vi "ACDC_Config.vi"(8 "error in (no error)":errorcluster, 9 "Input Config Array":T1[](array[typedef])=[0, 0, 0, 0, 0, 0, 0, 0, 0, 0, 0, 0, 0, 0, 0, 0, 0, 0, 0, 0, 0, 0, 0, 0, 0, 0, 0, 0, 0, 0, 0, 0] items=["AC Coupled", "DC Coupled", "IEPE AC Coupled"], 10 "Data Rate [S/s]":u32) -> (0 "error out":errorcluster)   [LabVIEW 2017, in "BOP_VibAPI_8.lvlib"]
uses:
  <vilib>/addons/InsightCM/Devices/Shared/Cms/Fpga/Acquisition/source/subVIs/VibAPI_8/BOP_VibAPI_8.lvlib
  <vilib>/LabVIEW Targets/FPGA/cRIO/shared/nicrio_ModuleControls/nicrio_cRIO-9232_ConfigModeRing.ctl
  <vilib>/rvi/eio/common/nirviEmuTemplatePropertySet_errors.vi
  <vilib>/eio/EIOPropertyNode/EIOPropertyNode.xnode
  <vilib>/LabVIEW Targets/FPGA/cRIO/shared/nicrio_ModuleControls/nicrio_cRIO-9232_DataRatesRing2.ctl
  <vilib>/rvi/eio/common/nirviEmuTemplatePropertyGet_errors.vi
  <vilib>/rvi/eio/common/nirviEmuTemplatePropertyGet_noerrors.vi
  <vilib>/rvi/eio/common/nirviEmuTemplatePropertySet_noerrors.vi
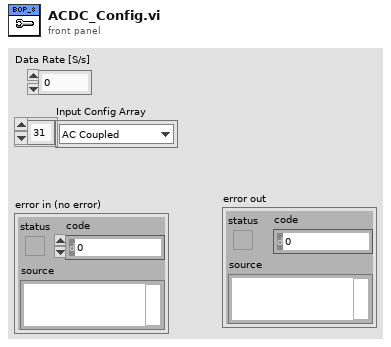
[diagram p1: front panel]
types:
  T1 = typedef "nicrio_cRIO-9232_ConfigModeRing.ctl" = u8
  T2 = typedef "nicrio_cRIO-9232_DataRatesRing2.ctl" = u8
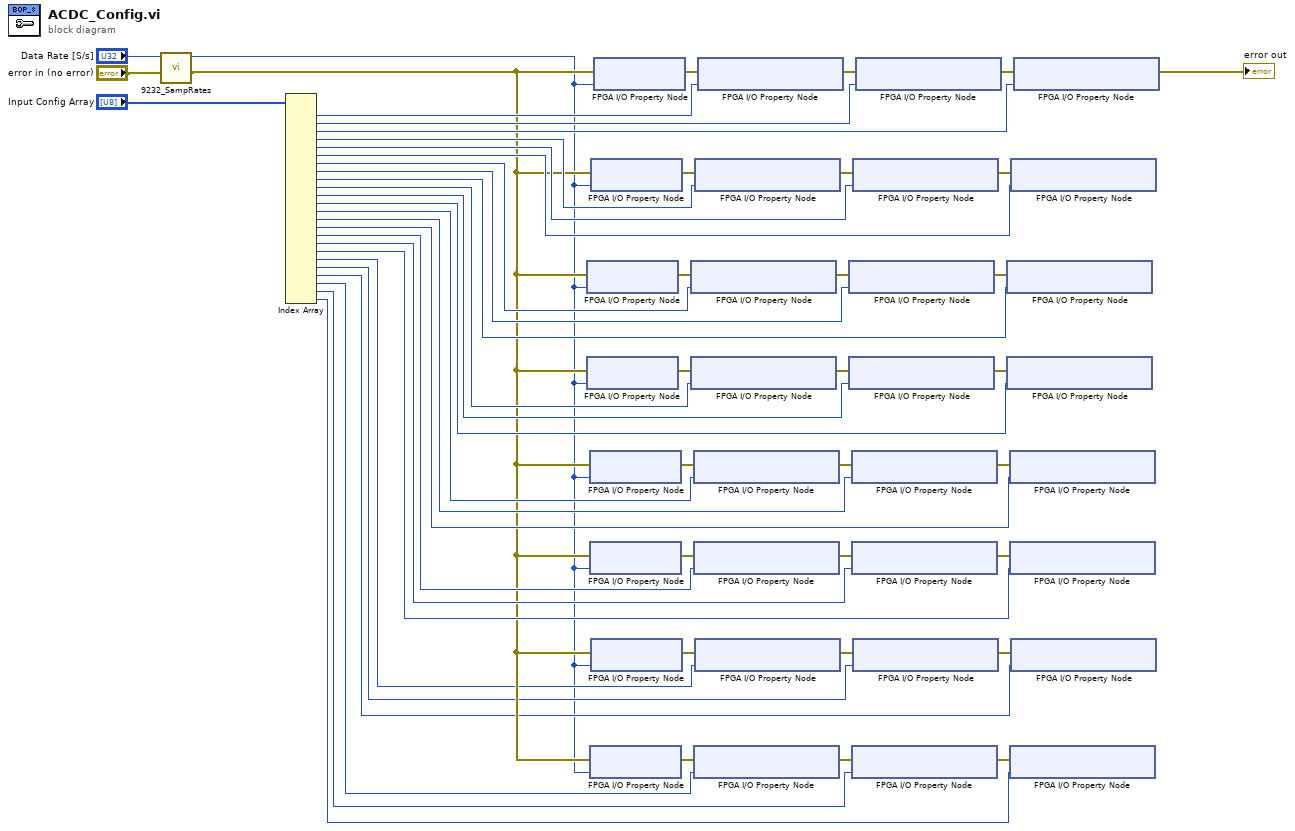
[diagram p0: block diagram]
diagram:
  n1 = call <vilib>:"9232_SampRates.vi"("error in (no error)"="error in (no error)", "Data Rate [S/s]"="Data Rate [S/s]") -> ("error out"=w8:errorcluster, "Data Rate"=w4:T2)  [unwired: 8 in]
  n2 = Index Array(array="Input Config Array") -> (element #1=w46:T1, element #2=w45:T1, element #3=w41:T1, element #4=w44:T1, element #5=w43:T1, element #6=w42:T1, element #7=w37:T1, element #8=w36:T1, element #9=w35:T1, element #10=w31:T1, element #11=w30:T1, element #12=w29:T1, element #13=w25:T1, element #14=w24:T1, element #15=w23:T1, element #16=w19:T1, element #17=w18:T1, element #18=w17:T1, element #19=w7:T1, element #20=w6:T1, element #21=w5:T1, element #22=w3:T1, element #23=w2:T1, element #24=w1:T1)  [unwired: 24 in]
  n3 = xnode "FPGA I/O Property Node"("error in"=w8, "Data Rate"=w4) -> ("error out"=w40:errorcluster)  [unwired: 1 in, 1 out]
  n4 = xnode "FPGA I/O Property Node"("error in"=w8, "Data Rate"=w4) -> ("error out"=w32:errorcluster)  [unwired: 1 in, 1 out]
  n5 = xnode "FPGA I/O Property Node"("error in"=w8, "Data Rate"=w4) -> ("error out"=w28:errorcluster)  [unwired: 1 in, 1 out]
  n6 = xnode "FPGA I/O Property Node"("error in"=w8, "Data Rate"=w4) -> ("error out"=w20:errorcluster)  [unwired: 1 in, 1 out]
  n7 = xnode "FPGA I/O Property Node"("error in"=w8, "Data Rate"=w4) -> ("error out"=w9:errorcluster)  [unwired: 1 in, 1 out]
  n8 = xnode "FPGA I/O Property Node"("error in"=w8, "Data Rate"=w4) -> ("error out"=w47:errorcluster)  [unwired: 1 in, 1 out]
  n9 = xnode "FPGA I/O Property Node"("error in"=w8, "Data Rate"=w4) -> ("error out"=w14:errorcluster)  [unwired: 1 in, 1 out]
  n10 = xnode "FPGA I/O Property Node"("error in"=w8, "Data Rate"=w4) -> ("error out"=w48:errorcluster)  [unwired: 1 in, 1 out]
  n11 = xnode "FPGA I/O Property Node"("error in"=w40, "Input Configuration"=w37) -> ("error out"=w39:errorcluster)  [unwired: 1 in, 1 out]
  n12 = xnode "FPGA I/O Property Node"("error in"=w32, "Input Configuration"=w31) -> ("error out"=w33:errorcluster)  [unwired: 1 in, 1 out]
  n13 = xnode "FPGA I/O Property Node"("error in"=w28, "Input Configuration"=w25) -> ("error out"=w27:errorcluster)  [unwired: 1 in, 1 out]
  n14 = xnode "FPGA I/O Property Node"("error in"=w20, "Input Configuration"=w19) -> ("error out"=w21:errorcluster)  [unwired: 1 in, 1 out]
  n15 = xnode "FPGA I/O Property Node"("error in"=w9, "Input Configuration"=w3) -> ("error out"=w10:errorcluster)  [unwired: 1 in, 1 out]
  n16 = xnode "FPGA I/O Property Node"("error in"=w47, "Input Configuration"=w44) -> ("error out"=w51:errorcluster)  [unwired: 1 in, 1 out]
  n17 = xnode "FPGA I/O Property Node"("error in"=w14, "Input Configuration"=w7) -> ("error out"=w13:errorcluster)  [unwired: 1 in, 1 out]
  n18 = xnode "FPGA I/O Property Node"("error in"=w48, "Input Configuration"=w46) -> ("error out"=w49:errorcluster)  [unwired: 1 in, 1 out]
  n19 = xnode "FPGA I/O Property Node"("error in"=w39, "Input Configuration"=w36) -> ("error out"=w38:errorcluster)  [unwired: 1 in, 1 out]
  n20 = xnode "FPGA I/O Property Node"("error in"=w33, "Input Configuration"=w30) -> ("error out"=w34:errorcluster)  [unwired: 1 in, 1 out]
  n21 = xnode "FPGA I/O Property Node"("error in"=w27, "Input Configuration"=w24) -> ("error out"=w26:errorcluster)  [unwired: 1 in, 1 out]
  n22 = xnode "FPGA I/O Property Node"("error in"=w21, "Input Configuration"=w18) -> ("error out"=w22:errorcluster)  [unwired: 1 in, 1 out]
  n23 = xnode "FPGA I/O Property Node"("error in"=w10, "Input Configuration"=w2) -> ("error out"=w11:errorcluster)  [unwired: 1 in, 1 out]
  n24 = xnode "FPGA I/O Property Node"("error in"=w51, "Input Configuration"=w43) -> ("error out"=w52:errorcluster)  [unwired: 1 in, 1 out]
  n25 = xnode "FPGA I/O Property Node"("error in"=w13, "Input Configuration"=w6) -> ("error out"=w12:errorcluster)  [unwired: 1 in, 1 out]
  n26 = xnode "FPGA I/O Property Node"("error in"=w49, "Input Configuration"=w45) -> ("error out"=w50:errorcluster)  [unwired: 1 in, 1 out]
  n27 = xnode "FPGA I/O Property Node"("error in"=w38, "Input Configuration"=w35) -> ()  [unwired: 1 in, 2 out]
  n28 = xnode "FPGA I/O Property Node"("error in"=w34, "Input Configuration"=w29) -> ()  [unwired: 1 in, 2 out]
  n29 = xnode "FPGA I/O Property Node"("error in"=w26, "Input Configuration"=w23) -> ()  [unwired: 1 in, 2 out]
  n30 = xnode "FPGA I/O Property Node"("error in"=w22, "Input Configuration"=w17) -> ()  [unwired: 1 in, 2 out]
  n31 = xnode "FPGA I/O Property Node"("error in"=w11, "Input Configuration"=w1) -> ()  [unwired: 1 in, 2 out]
  n32 = xnode "FPGA I/O Property Node"("error in"=w52, "Input Configuration"=w42) -> ()  [unwired: 1 in, 2 out]
  n33 = xnode "FPGA I/O Property Node"("error in"=w12, "Input Configuration"=w5) -> ()  [unwired: 1 in, 2 out]
  n34 = xnode "FPGA I/O Property Node"("error in"=w50, "Input Configuration"=w41) -> ("error out"=→"error out":errorcluster)  [unwired: 1 in, 1 out]
